vi "BLE_Write_Without_Response.vi"(0 ".NET Refnum in":refnum<k24>, 5 "UUID":string, 7 "WriteByteArray":u8[](array[numeric]), 11 "error in (no error)":errorcluster) -> (4 ".NET Refnum out":refnum<k24>, 10 "Result":string, 15 "error out":errorcluster)   [LabVIEW 2020, in "BLE.lvlib"]
uses:
  C:/Users/Trait/Desktop/LabView Project/LabView BLE DataACQ/BLELib.dll
  BLELib.dll
  BLE.lvlib
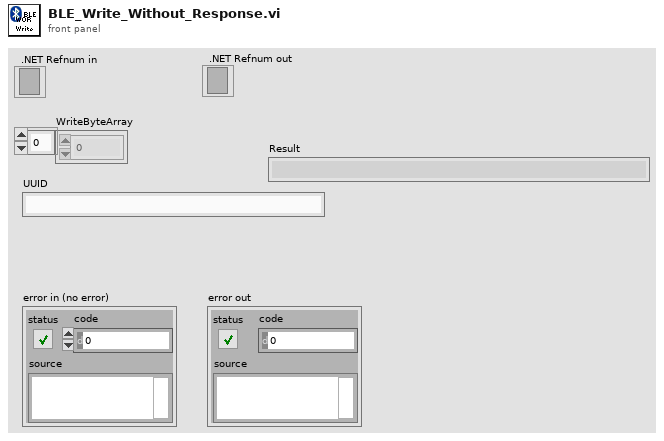
[diagram p1: front panel]
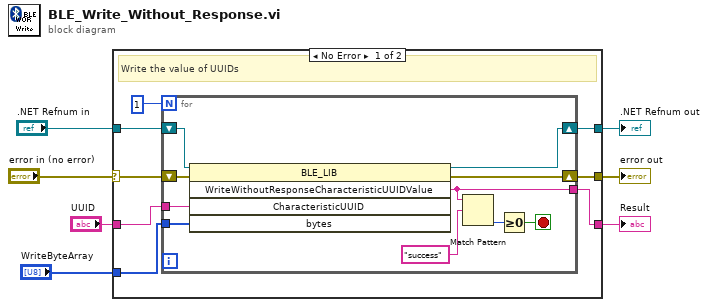
[diagram p0: block diagram]
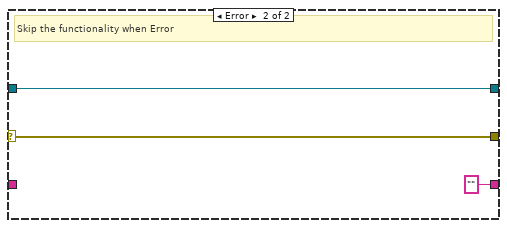
[diagram p2: hidden frame]
diagram:
  n1 = case shown="No Error" "error in (no error)" {
    selector: "error in (no error)" -> [w12 w28]
    tunnel: "UUID" -> [w15 _]
    tunnel: "WriteByteArray" -> [w14 _]
    tunnel: [w13 "" ("Result")] -> w5
    tunnel: [w11 w28] -> w3
    tunnel: [w10 w27] -> w2
    tunnel: ".NET Refnum in" -> [w9 w27]
    frame No Error {
      # "Write the value of UUIDs"
      n2 = for {
        N: 1 -> [_]
        tunnel: w15 -> [w25]
        tunnel: w14 -> [w16]
        tunnel: [w24] -> w13
        shift-right: [w22] -> w11
        shift-left: w12 -> [w23]
        shift-right: [w21] -> w10
        shift-left: w9 -> [w20]
        stop <- w17 stop-if-true
        n3 = invoke class="BLE_LIB" method="WriteWithoutResponseCharacteristicUUIDValue"(reference=w20, error in=w23, "CharacteristicUUID"=w25, "bytes"=w16) -> (reference out=w21:refnum<k24>, error out=w22:errorcluster, "WriteWithoutResponseCharacteristicUUIDValue"=w24:string)  [unwired: 1 in, 2 out]
        n4 = Match Pattern(string=w24, regular expression="success") -> (offset past match=w18:i32)  [unwired: 1 in, 3 out]
        n5 = Greater Or Equal To 0?(x=w18) -> (x >= 0?=w17:bool)
      }
    }
    frame Error {
      # "Skip the functionality when Error"
    }
  }
  "Result" <- w5
  "error out" <- w3
  ".NET Refnum out" <- w2
